vi "Read Total Flow.vi"(8 "error in (no error)":errorcluster, 11 "VISA resource name":refnum<visa-resource-name>) -> (0 "error out":errorcluster, 2 "Total Flow":dbl, 3 "VISA resource name out":refnum<visa-resource-name>)   [LabVIEW 2023, in "Fluke Molbox 1 Plus.lvlib"]
doc: "Reads the total current mass or volume flowed over a set period. This requires starting a totalizing cycle. \n\n<B>Note:</B>\nUse \"Query Cycle Progress\" to see if the Totalize cycle has completed."
uses:
  Fluke Molbox 1 Plus.lvlib
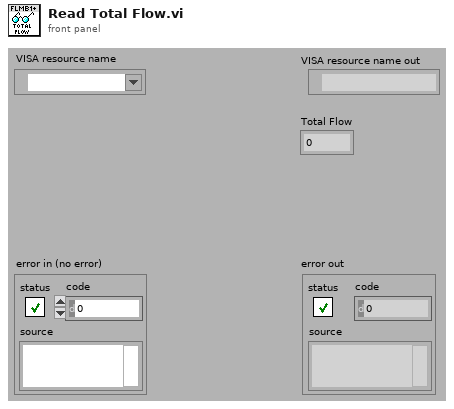
[diagram p1: front panel]
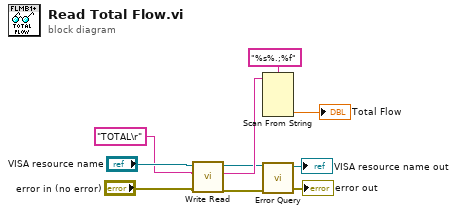
[diagram p0: block diagram]
diagram:
  n1 = call "Write Read.vi"("error in (no error)"="error in (no error)", "Write String"="TOTAL\r" ("write buffer"), "VISA resource name"="VISA resource name") -> ("error out"=w2:errorcluster, "Read Response"=w5:string, "VISA resource name out"=w1:refnum<visa-resource-name>)  [unwired: 6 in]
  n2 = Scan From String(format string="%s%.;%f", input string=w5) -> (output 2=→"Total Flow":dbl)  [unwired: 5 in, 3 out]
  n3 = call "Error Query.vi"("error in (no error)"=w2, "VISA resource name"=w1) -> ("error out"=→"error out":errorcluster, "VISA resource name out"=→"VISA resource name out":refnum<visa-resource-name>)  [unwired: 6 in, 2 out]
